vi "Create Wheel.vi"   [LabVIEW 2017, in "NI_Robotics_Wheel.lvclass"]
doc: "Creates a wheel of the type you specify that you can add to a steering frame. You must manually select the polymorphic instance to use."
uses:
  <vilib>/robotics/Steering/Wheel/NI_Robotics_Wheel.lvclass
  <vilib>/robotics/Steering/Fixed Wheel/NI_Robotics_Fixed Wheel.lvclass
  <vilib>/robotics/Steering/Steering Wheel/NI_Robotics_Steering Wheel.lvclass
  <vilib>/robotics/Steering/Caster Wheel/NI_Robotics_Caster Wheel.lvclass
  <vilib>/robotics/Steering/Mecanum Wheel/NI_Robotics_Mecanum Wheel.lvclass
  <vilib>/robotics/Steering/Omnidirectional Wheel/NI_Robotics_Omnidirectional Wheel.lvclass
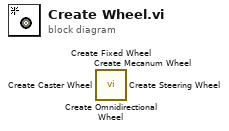
[diagram p0: block diagram]
diagram:
  n1 = call <vilib>:"Create Omnidirectional Wheel.vi"() -> ()  [unwired: 10 in, 2 out]
  n2 = call <vilib>:"Create Mecanum Wheel.vi"() -> ()  [unwired: 10 in, 2 out]
  n3 = call <vilib>:"Create Caster Wheel.vi"() -> ()  [unwired: 10 in, 2 out]
  n4 = call <vilib>:"Create Steering Wheel.vi"() -> ()  [unwired: 10 in, 2 out]
  n5 = call <vilib>:"Create Fixed Wheel.vi"() -> ()  [unwired: 10 in, 2 out]
